vi "CSTK_QD_Enum Creator.vi"(6 "Variant in":variant, 7 "Shift Pressed?":bool, 8 "error in (no error)":errorcluster, 10 "QD Combo Box Ref":refnum<vi>, 11 "QD Launch VI Ref":refnum<vi>) -> (0 "error out":errorcluster, 4 "Variant out":variant)   [LabVIEW 2015]
doc: "打开Enum编辑器\n\n默认快捷键 - [E]"
uses:
  Library/Enum Creator/CSTK_Enum Creator.lvlib
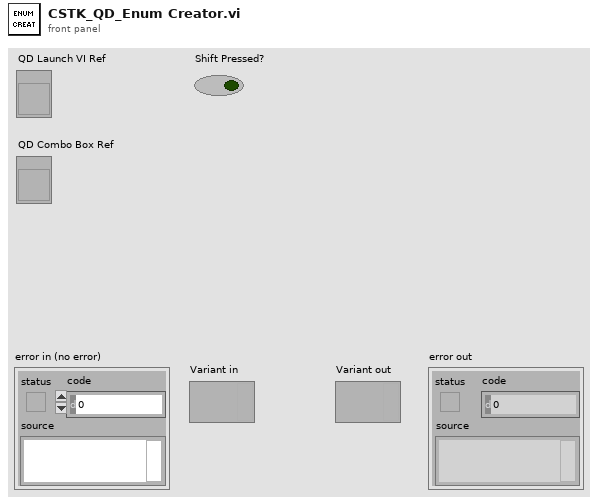
[diagram p1: front panel]
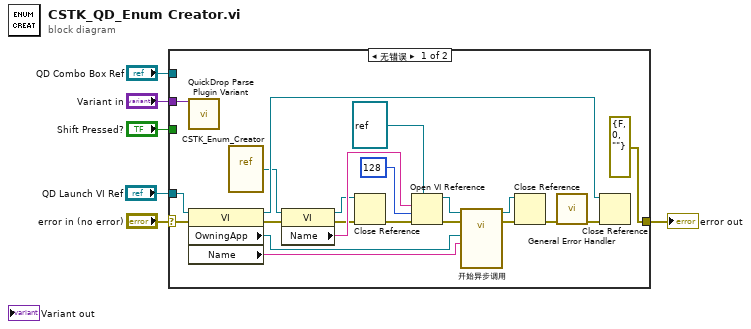
[diagram p0: block diagram]
diagram:
  n1 = case shown="无错误" "error in (no error)" {
    selector: "error in (no error)" -> [w18 w28]
    tunnel: [errorcluster {"status"=FALSE, "code"=0, "source"=""} ("错误常量") w28] -> w5
    tunnel: "QD Launch VI Ref" -> [w19 _]
    tunnel: "Shift Pressed?" -> [_ _]
    tunnel: "QD Combo Box Ref" -> [_ _]
    tunnel: "Variant in" -> [w27 _]
    frame No Error {
      n2 = call <vilib>:"QuickDrop Parse Plugin Variant.vi"("QDKS Variant in"=w27) -> ()  [unwired: 12 in, 3 out]
      n3 = property class="VI"(reference=w19, error in=w18) -> (reference out=w13:refnum<vi>, error out=w15:errorcluster, "OwningApp"=w17:refnum<vi>, "Name"=w16:string)
      n4 = vi-ref "CSTK_Enum_Creator.vi"() -> (w7:refnum<vi>)
      n5 = property class="VI"(reference=w7, error in=w15) -> (reference out=w9:refnum<vi>, error out=w10:errorcluster, "Name"=w20:string)
      n6 = Close Reference(reference=w9, error in (no error)=w10) -> (error out=w8:errorcluster)
      n7 = Open VI Reference(type specifier VI Refnum (for type only)=refnum<vi> refnum ("类型说明符VI引用句柄（仅用于类型）"), vi path=w20, options=128 ("选项"), error in (no error)=w8) -> (vi reference=w21:refnum<vi>, error out=w22:errorcluster)  [unwired: 2 in]
      n8 = call-by-ref "开始异步调用"(reference=w21, error in=w22, "应用程序:菜单启动:VI"=w16, "应用程序引用（本地）"=w17) -> (reference out=w23:refnum<vi>, error out=w24:errorcluster)  [unwired: 10 in]
      n9 = Close Reference(reference=w23, error in (no error)=w24) -> (error out=w14:errorcluster)
      n10 = call <vilib>:"General Error Handler.vi"("error in (no error)"=w14) -> ("error out"=w12:errorcluster)  [unwired: 10 in, 4 out]
      n11 = Close Reference(reference=w13, error in (no error)=w12) -> ()  [unwired: 1 out]
    }
    frame Error {
    }
  }
  "error out" <- w5
